vi "ReportPart_A131258.vi"(6 "试验项目":enum32{"压装"}(ring), 8 "error in":errorcluster, 9 "索引":i32, 10 "合格":T1, 11 "report in":refnum<class "NI_report.lvclass">) -> (0 "error out 2":errorcluster caption="error out", 3 "report out":refnum<class "NI_report.lvclass">)   [LabVIEW 2020]
uses:
  <vilib>/Utility/NIReport.llb/image depth.ctl
  <vilib>/Utility/NIReport.llb/NI_ReportGenerationCore.lvlib
  <vilib>/Utility/NIReport.llb/NI_report.lvclass
  <vilib>/Utility/NIReport.llb/Append Report Text (str wrap).vi
  <vilib>/Utility/NIReport.llb/Word/NI_Word.lvclass
  <vilib>/addons/_office/NI_ReportGenerationToolkit.lvlib
  <vilib>/addons/_office/word.llb/Word Easy Table (str).vi
  <vilib>/addons/_office/_exclsub.llb/font.ctl
  Global_Variable/Global.vi
  Global_Variable/A131258.vi
  OK.ctl
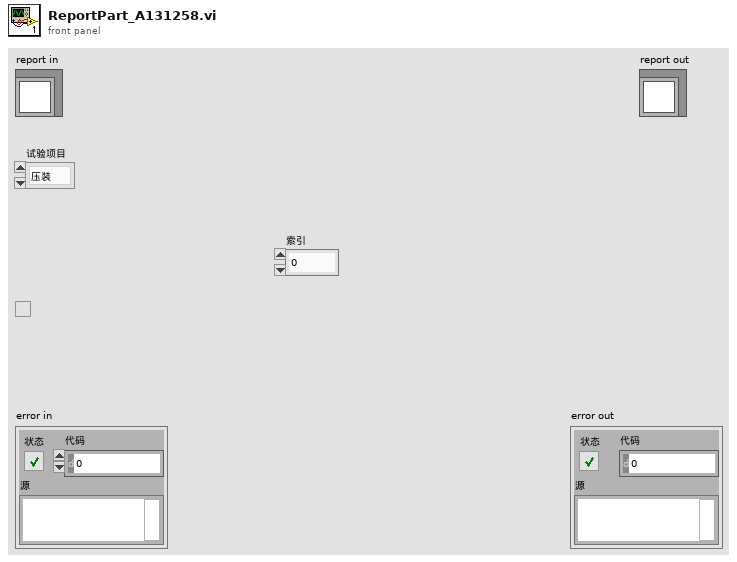
[diagram p1: front panel]
types:
  T1 = typedef "OK.ctl" = bool
  T2 = cluster{"Charset (-1)":i16, "Weight (-1)":i16, "Name":string, "Size":string}
  T3 = cluster{"Italic":enum16{"Italic Unchanged", "Italic On", "Italic Off"}, "Strike Through":enum16{"Strike Through Unchanged", "Strike Through On", "Strike Through Off"}, "Underline":enum16{"Underline Unchanged", "Underline On", "Underline Off"}, "Bold":enum16{"Bold Unchanged", "Bold On", "Bold Off"}}
  T4 = typedef "NI_ReportGenerationToolkit.lvlib/font.ctl" = cluster{"font name":string, "font size":dbl, "bold":u16, "italic":u16, "underline":u16, "strike through":u16, "font color":u32}
  T5 = typedef "NI_ReportGenerationCore.lvlib/image depth.ctl" = u16
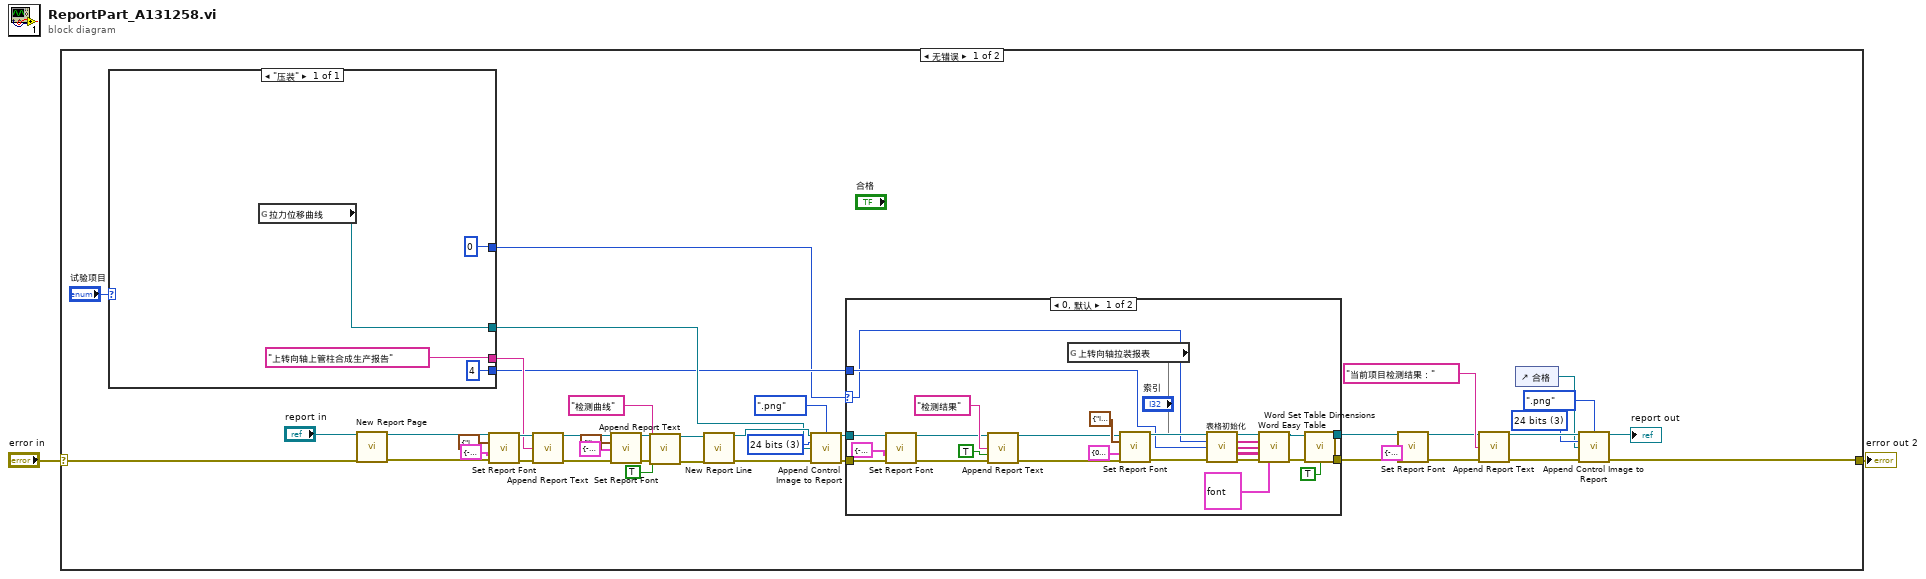
[diagram p0: block diagram]
diagram:
  n1 = case shown="无错误" "error in" {
    selector: "error in" -> [w22 w77]
    tunnel: [w16 w77] -> w1
    frame No Error {
      w14 = T5 3 items=["B&W", "4 bits", "8 bits", "24 bits"] ("image depth")
      w42 = T5 3 items=["B&W", "4 bits", "8 bits", "24 bits"] ("image depth")
      n2 = case shown="\"压装\"" "试验项目" {
        tunnel: [w73] -> w5
        tunnel: ["上转向轴上管柱合成生产报告" ("text")] -> w36
        tunnel: [4 ("长度")] -> w4
        tunnel: [0 ("长度")] -> w3
        frame "压装" {
          n3 = global read "A131258.vi" "拉力位移曲线"() -> (w73:refnum<vi>)
        }
      }
      n4 = call-dynamic "New Report Page.vi"("report in"="report in", "error in (no error)"=w22) -> ("report out"=w20:refnum<class "NI_report.lvclass">, "error out"=w21:errorcluster)  [unwired: 12 in]
      n5 = call-dynamic "Set Report Font.vi"("report in"=w20, "text options"=T3 {"Italic"=enum."Italic Unchanged", "Strike Through"=enum."Strike Through Unchanged", "Underline"=enum."Underline Unchanged", "Bold"=enum."Bold On"}, "font settings"=T2 {"Charset (-1)"=-1, "Weight (-1)"=-1, "Name"="楷体", "Size"="16 "}, "error in (no error)"=w21) -> ("report out"=w41:refnum<class "NI_report.lvclass">, "error out"=w40:errorcluster)  [unwired: 9 in, 1 out]
      n6 = call-poly <vilib>:"Append Report Text.vi"("report in"=w41, "text"=w36, "error in (no error)"=w40) -> ("report out"=w33:refnum<class "NI_report.lvclass">, "error out"=w32:errorcluster)  [unwired: 9 in, 2 out]
      n7 = call-dynamic "Set Report Font.vi"("report in"=w33, "text options"=T3 {"Italic"=enum."Italic Unchanged", "Strike Through"=enum."Strike Through Unchanged", "Underline"=enum."Underline Unchanged", "Bold"=enum."Bold Off"}, "font settings"=T2 {"Charset (-1)"=-1, "Weight (-1)"=-1, "Name"="宋体", "Size"="12 "}, "error in (no error)"=w32) -> ("report out"=w29:refnum<class "NI_report.lvclass">, "error out"=w26:errorcluster)  [unwired: 9 in, 1 out]
      n8 = call-poly <vilib>:"Append Report Text.vi"("report in"=w29, "text"="检测曲线", "append on new line? (F)"=TRUE, "error in (no error)"=w26) -> ("report out"=w28:refnum<class "NI_report.lvclass">, "error out"=w27:errorcluster)  [unwired: 8 in, 2 out]
      n9 = call-dynamic "New Report Line.vi"("report in"=w28, "error in (no error)"=w27) -> ("report out"=w43:refnum<class "NI_report.lvclass">, "error out"=w44:errorcluster)  [unwired: 12 in]
      n10 = call-dynamic "Append Control Image to Report.vi"("report in"=w43, "image file type (.jpg)"=enum16{".jpg", ".png"}.".png", "image depth"=w42, "ctrl reference"=w5, "error in (no error)"=w44) -> ("report out"=w38:refnum<class "NI_report.lvclass">, "error out"=w37:errorcluster)  [unwired: 7 in, 2 out]
      n11 = case shown="0, 默认" w3 {
        selector: w3 -> [w45 _]
        tunnel: w38 -> [w66 w72]
        tunnel: w37 -> [w64 w71]
        tunnel: [w51 w72] -> w7
        tunnel: [w50 w71] -> w6
        tunnel: w4 -> [w46 _]
        frame 0, Default {
          n12 = call-dynamic "Set Report Font.vi"("report in"=w66, "font settings"=T2 {"Charset (-1)"=-1, "Weight (-1)"=-1, "Name"="宋体", "Size"="12 "}, "error in (no error)"=w64) -> ("report out"=w67:refnum<class "NI_report.lvclass">, "error out"=w65:errorcluster)  [unwired: 10 in, 1 out]
          n13 = call-poly <vilib>:"Append Report Text.vi"("report in"=w67, "text"="检测结果", "append on new line? (F)"=TRUE, "error in (no error)"=w65) -> ("report out"=w49:refnum<class "NI_report.lvclass">, "error out"=w48:errorcluster)  [unwired: 8 in, 2 out]
          n14 = global read "Global.vi" "上转向轴拉装报表"() -> (w47)
          n15 = call-dynamic "Set Report Font.vi"("report in"=w49, "text options"=T3 {"Italic"=enum."Italic Unchanged", "Strike Through"=enum."Strike Through Unchanged", "Underline"=enum."Underline Unchanged", "Bold"=enum."Bold Unchanged"}, "font settings"=T2 {"Charset (-1)"=0, "Weight (-1)"=-1, "Name"="微软雅黑", "Size"="12 "}, "error in (no error)"=w48) -> ("report out"=w53:refnum<class "NI_report.lvclass">, "error out"=w52:errorcluster)  [unwired: 9 in, 1 out]
          n16 = call "表格初始化.vi"("表格引用"=w47, "索引"=w45, "长度"=w46, "错误输入（无错误）"=w52) -> ("行首字符串[]"=w55:string[], "列首字符串[]"=w54:string[], "文本数据"=w57:string[][], "错误输出"=w60:errorcluster)  [unwired: 7 in, 1 out]
          n17 = call-poly <vilib>:"Word Easy Table.vi"("report in"=w53, "row headers"=w55, "column headers"=w54, "data"=w57, "error in (no error)"=w60, "font"=T4 {"font name"="宋体", "font size"=12.0, "bold"=2, "italic"=2, "underline"=2, "strike through"=2, "font color"=16777216}) -> ("report out"=w58:refnum<class "NI_report.lvclass">, "error out"=w59:errorcluster)  [unwired: 7 in, 1 out]
          n18 = call <vilib>:"Word Set Table Dimensions.vi"("report in"=w58, "error in (no error)"=w59, "fit to page width? (F)"=TRUE) -> ("report out"=w51:refnum<class "NI_report.lvclass">, "error out"=w50:errorcluster)  [unwired: 11 in]
        }
        frame -1 {
        }
      }
      n19 = call-dynamic "Set Report Font.vi"("report in"=w7, "font settings"=T2 {"Charset (-1)"=-1, "Weight (-1)"=-1, "Name"="宋体", "Size"="16 "}, "error in (no error)"=w6) -> ("report out"=w11:refnum<class "NI_report.lvclass">, "error out"=w12:errorcluster)  [unwired: 10 in, 1 out]
      n20 = call-poly <vilib>:"Append Report Text.vi"("report in"=w11, "text"="当前项目检测结果：", "error in (no error)"=w12) -> ("report out"=w19:refnum<class "NI_report.lvclass">, "error out"=w17:errorcluster)  [unwired: 9 in, 2 out]
      n21 = control-ref of="合格"() -> (w13:refnum<vi>)
      n22 = call-dynamic "Append Control Image to Report.vi"("report in"=w19, "image file type (.jpg)"=enum16{".jpg", ".png"}.".png", "image depth"=w14, "ctrl reference"=w13, "error in (no error)"=w17) -> ("report out"=→"report out":refnum<class "NI_report.lvclass">, "error out"=w16:errorcluster)  [unwired: 7 in, 2 out]
    }
    frame Error {
    }
  }
  "error out 2" <- w1
